vi "server.vi"() -> ()   [LabVIEW 2014, in "Experiment.lvclass"]
uses:
  Experiment.lvclass
  HSDIO/HSDIO_settings.ctl
  <instrlib>/niHSDIO/niHSDIO.llb/niHSDIO_ctl Trigger Script - trigID Values (Ring).ctl
  <instrlib>/niHSDIO/niHSDIO.llb/niHSDIO_ctl Trigger Source Values (Ring).ctl
  <instrlib>/niHSDIO/niHSDIO.llb/niHSDIO_ctl Trigger DigEdge - Edge Values (Ring).ctl
  <instrlib>/niHSDIO/niHSDIO.llb/niHSDIO_ctl Trigger DigLvl - Level Values (Ring).ctl
  HSDIO/waveform.ctl
  Camera/Hamamatsu_C9100-13/camera_setup.ctl
  states.ctl
  Analog_output/AO_settings.ctl
  DAQmx_DO/settings.ctl
  Analog_Input/settings.ctl
  Counter/Counter_Settings_Control.ctl
  <vilib>/Platform/TimedLoop/XDataNode/timing_clust.ctl
  <vilib>/Platform/TimedLoop/XDataNode/nitl_modes.ctl
  <vilib>/Platform/TimedLoop/XDataNode/wakeup.ctl
  Experiment.lvclass/Experiment.ctl
  Globals.vi
  <vilib>/platform/TimedLoop/XDataNode/XDataNode.xnode
  HSDIO/HSDIO.lvclass
  DAQmx_DO/DAQmx_DO.lvclass
  Analog_output/Analog_Output.lvclass
  Analog_Input/Analog_Input.lvclass
  Counter/Counter.lvclass
  Camera/Hamamatsu_C9100-13/Hamamatsu_C9100-13.lvclass
  TCP_IP/TCP_IP.lvclass
  <vilib>/Platform/TimedLoop/XDataNode/XDNodeRunTimeDep.lvlib
panel:
  in  "IP address to listen on\n(blank to allow all networks)":string
  out "cycleContinuously":bool
  out "state":T1
  in  "port":u16=9000
  out "Loops while waiting for measurement isDone?":i32
  out "Log History":string
  in  "Tab Control":T2(tab)
  out "Measurement Timeout (ms)":u32=1
  out "HSDIO Settings":T3={"Enable HSDIO Pulses"=FALSE, "Clock Rate"=20000000.0, "Array of Script Triggers"=[], "Pulse Generation Script"="script script1\n     wait 1\nend script", "Start Trigger"={"Wait for start trigger?"=FALSE, "source (PFI 0)"="PFI0", "edge (rising)"=12, "description"=""}, "Hardware alignment quantum\n(in samples)"=1, "Array of Waveforms"=[], "description"="", "Resource Names"=[], "Active Channels"=[], "Initial States"=[], "Idle States"=[]} {"Hardware alignment quantum\n(in samples)" min=1 step=1; "Array of Script Triggers"."level" items=["High Level"=34, "Low Level"=35]; "Array of Script Triggers"."edge" items=["Rising Edge"=12, "Falling Edge"=13]; "Start Trigger"."edge (rising)" items=["Rising Edge"=12, "Falling Edge"=13]; "Clock Rate" min=0.0 max=200000000.0 format="%.2p"}
  out "Camera Setup":T9={"Analog Gain (0-5)"=0, "Exposure Time"=0.05, "EM Gain (0-255)"=0, "Trigger Polarity"="ATP P", "External Trigger Mode"="EMD L", "Scan Speed"="SSP H", "External Trigger Source"="ESC B", "Scan Mode"="SMD N", "Super Pixel Binning\n(if enabled in Scan Mode)"="1x1", "Camera Sub-array acquisition region\n(if enabled in scan mode)"={"Left"=0, "Top"=0, "Width"=512, "Height"=512}, "Use camera?"=FALSE, "# image buffers"=10, "shots per measurement"=2, "Force images to U16"=FALSE, "Low Light Sensitivity"="LLS 0", "cooling"="CSW F", "fan"="FAN F", "Frame Grabber acquisition region"={"Left"=0, "Top"=0, "Right"=512, "Bottom"=512}} {"Frame Grabber acquisition region"."Bottom" max=512 step=1; "Frame Grabber acquisition region"."Right" max=512 step=1; "Frame Grabber acquisition region"."Top" max=512 step=1; "Frame Grabber acquisition region"."Left" max=512 step=1; "shots per measurement" min=0 step=1; "# image buffers" min=0 step=1; "Camera Sub-array acquisition region\n(if enabled in scan mode)"."Height" min=16 max=512 step=16; "Camera Sub-array acquisition region\n(if enabled in scan mode)"."Width" min=16 max=512 step=16; "Camera Sub-array acquisition region\n(if enabled in scan mode)"."Top" max=496 step=16; "Camera Sub-array acquisition region\n(if enabled in scan mode)"."Left" max=496 step=16; "Analog Gain (0-5)" max=5 step=1}
  out "Analog Output Parameters":T10={"Enable Analog Out?"=FALSE, "Physical Channel"="PXI1Slot2/ao0:2", "Minimum Value"=-10.0, "Maximum Value"=10.0, "Samples per second"=0.0, "Start Trigger"={"Wait for start trigger?"=FALSE, "source"="/Dev1/PFI0", "edge"=10280}, "Analog Output Waveforms (channel, time)"=[], "Export trigger"={"Export Start Trigger?"=FALSE, "output terminal"=""}, "External Clock"={"Use external clock?"=FALSE, "source"="", "max expected clock rate"=200000000.0}} {"External Clock"."max expected clock rate" format="%#_13g"; "Start Trigger"."edge" items=["Rising"=10280, "Falling"=10171]; "Maximum Value" format="%0.2f"; "Minimum Value" format="%0.2f"}
  out "settings":T11={"enable"=FALSE, "samples_per_measurement"=1, "sample rate (Hz)"=-10.0, "source"="Dev3/ai0:2", "Start Trigger"={"Wait for start trigger?"=FALSE, "source"="/Dev1/PFI0", "edge"=10280}, "ground_mode"=""} {"Start Trigger"."edge" items=["Rising"=10280, "Falling"=10171]}
  out "DAQmx Pulse Settings":T12={"Enable DAQmx Pulses"=FALSE, "DAQmx Physical Channels"="Dev2/port0_32", "Clock Rate"=10000000.0, "units/sec (ms=1000)"=1000.0, "Start Trigger"={"Wait for start trigger?"=FALSE, "source"="/Dev1/PFI0", "edge"=10280}, "waveform"={"name"="", "transitions"=[], "states"=[]}} {"Start Trigger"."edge" items=["Rising"=10280, "Falling"=10171]; "Clock Rate" min=0.0 max=200000000.0 format="%.2p"}
  out "Counter Settings":T13 {"Array of Counter Settings"."clock rate (Hz)" format="%0.2f"}
  in  "Clear Log":bool
  in  "Return fake test data":bool
  out "Done":bool=TRUE
  in  "Restart":bool
  out "Log":string
  in  "Stop":bool
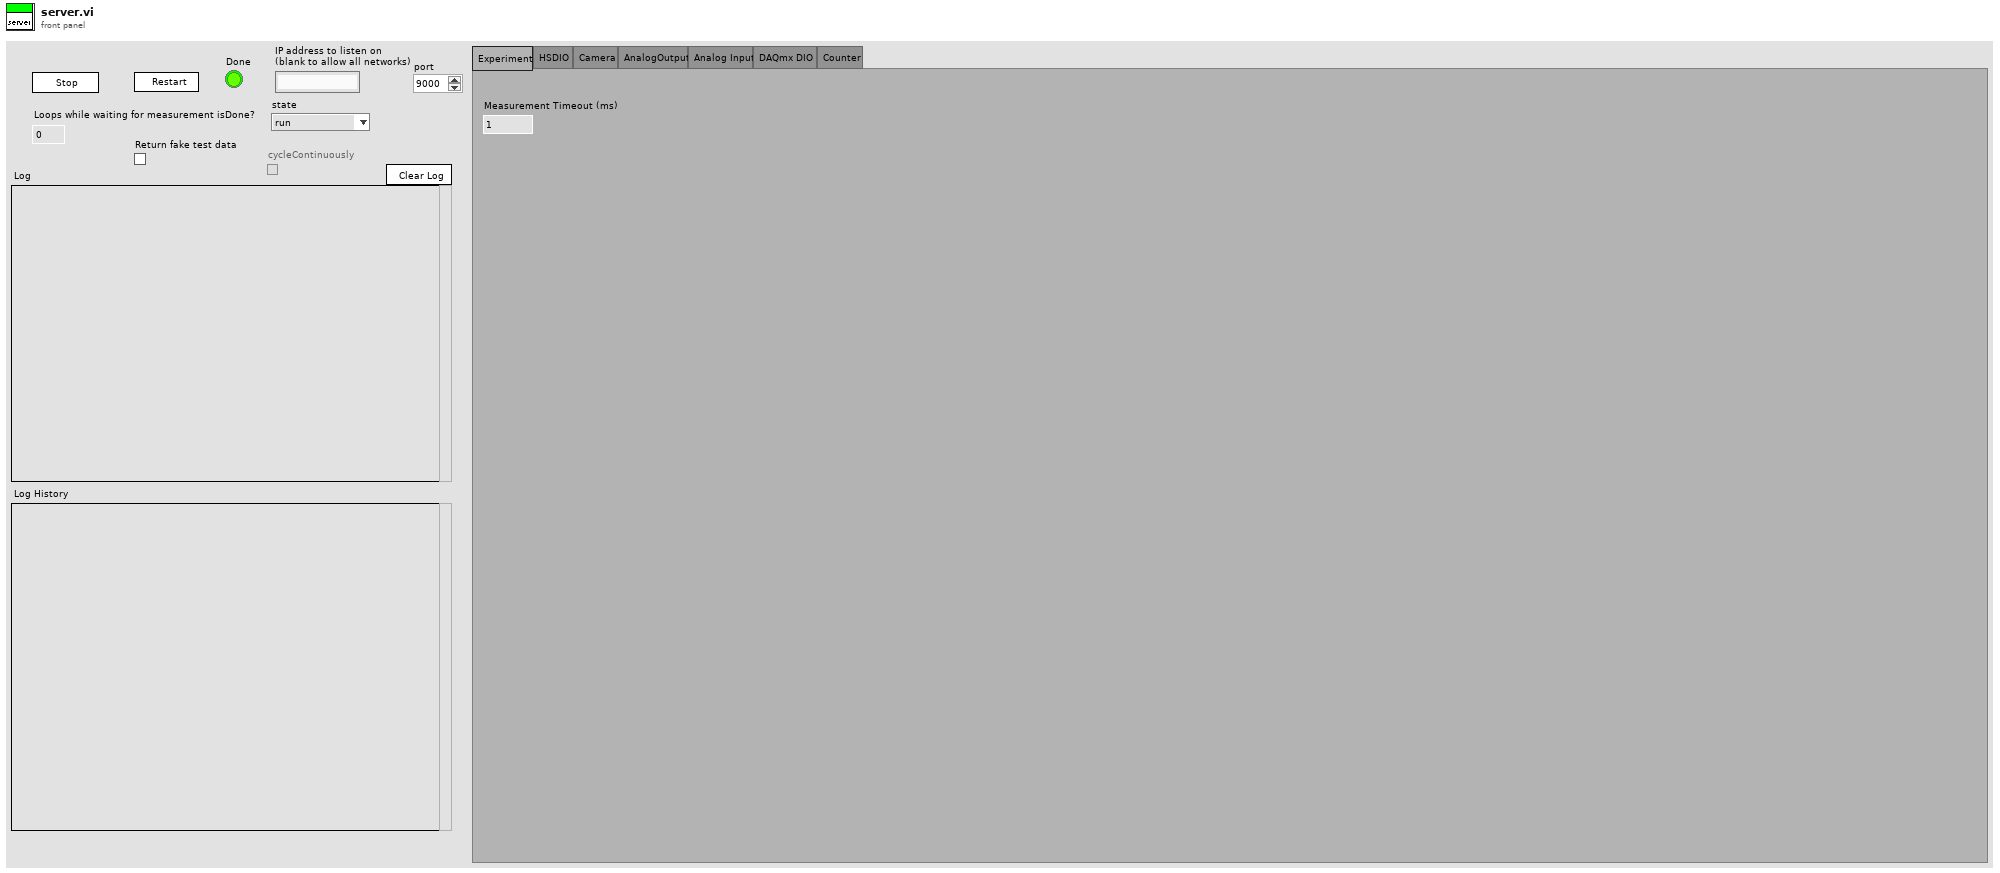
[diagram p1: front panel]
types:
  T1 = typedef "Experiment.lvclass/states.ctl" = enum16{"run", "pause", "shutdown gracefully", "halt immediately", "waiting for connection", "waiting for command"}
  T2 = enum32{"Experiment", "HSDIO", "Camera", "AnalogOutput", "Analog Input", "DAQmx DIO", "Counter"}
  T3 = typedef "HSDIO.lvclass/HSDIO_settings.ctl" = cluster{"Enable HSDIO Pulses":bool, "Clock Rate":dbl, "Array of Script Triggers":cluster{"trigger id (script trigger 0)":T4, "source (PFI 0)":T5, "Trigger Type":enum32{"Edge", "Level"}, "edge":T6, "level":T7}[], "Pulse Generation Script":string, "Start Trigger":cluster{"Wait for start trigger?":bool, "source (PFI 0)":T5, "edge (rising)":T6, "description":string}, "Hardware alignment quantum\n(in samples)":u16, "Array of Waveforms":T8[], "description":string, "Resource Names":refnum<k15>[], "Active Channels":string[], "Initial States":string[], "Idle States":string[]}
  T4 = typedef "niHSDIO_ctl Trigger Script - trigID Values (Ring).ctl" = string
  T5 = typedef "niHSDIO_ctl Trigger Source Values (Ring).ctl" = string
  T6 = typedef "niHSDIO_ctl Trigger DigEdge - Edge Values (Ring).ctl" = i32
  T7 = typedef "niHSDIO_ctl Trigger DigLvl - Level Values (Ring).ctl" = i32
  T8 = typedef "HSDIO.lvclass/waveform.ctl" = cluster{"name":string, "transitions":u32[], "states":u8[][]}
  T9 = typedef "Hamamatsu_C9100-13.lvclass/camera_setup.ctl" = cluster{"Analog Gain (0-5)":u8, "Exposure Time":dbl, "EM Gain (0-255)":u8, "Trigger Polarity":string, "External Trigger Mode":string, "Scan Speed":string, "External Trigger Source":string, "Scan Mode":string, "Super Pixel Binning\n(if enabled in Scan Mode)":string, "Camera Sub-array acquisition region\n(if enabled in scan mode)":cluster{"Left":u16, "Top":u16, "Width":u16, "Height":u16}, "Use camera?":bool, "# image buffers":i32, "shots per measurement":i32, "Force images to U16":bool, "Low Light Sensitivity":string, "cooling":string, "fan":string, "Frame Grabber acquisition region":cluster{"Left":i32, "Top":i32, "Right":i32, "Bottom":i32}}
  T10 = typedef "Analog_Output.lvclass/AO_settings.ctl" = cluster{"Enable Analog Out?":bool, "Physical Channel":tag, "Minimum Value":dbl, "Maximum Value":dbl, "Samples per second":dbl, "Start Trigger":cluster{"Wait for start trigger?":bool, "source":tag, "edge":i32}, "Analog Output Waveforms (channel, time)":dbl[][], "Export trigger":cluster{"Export Start Trigger?":bool, "output terminal":tag}, "External Clock":cluster{"Use external clock?":bool, "source":tag, "max expected clock rate":dbl}}
  T11 = typedef "Analog_Input.lvclass/settings.ctl" = cluster{"enable":bool, "samples_per_measurement":i32, "sample rate (Hz)":dbl, "source":tag, "Start Trigger":cluster{"Wait for start trigger?":bool, "source":tag, "edge":i32}, "ground_mode":string}
  T12 = typedef "DAQmx_DO.lvclass/settings.ctl" = cluster{"Enable DAQmx Pulses":bool, "DAQmx Physical Channels":tag, "Clock Rate":dbl, "units/sec (ms=1000)":dbl, "Start Trigger":cluster{"Wait for start trigger?":bool, "source":tag, "edge":i32}, "waveform":T8}
  T13 = typedef "Counter.lvclass/Counter_Settings_Control.ctl" = cluster{"enable":bool, "Array of Counter Settings":cluster{"counter source":tag, "clock source":tag, "clock rate (Hz)":dbl}[]}
  T14 = typedef "XDNodeRunTimeDep.lvlib/timing_clust.ctl" = cluster{"Expected End [f-1]":u64, "Actual End [f-1]":u64, "Finished Late? [f-1]":bool, "Expected End [i-1]":u64, "Actual End [i-1]":u64, "Finished Late? [i-1]":bool, "Expected Start [i]":u64, "Actual Start [i]":u64, "Expected Start [f]":u64, "Actual Start [f]":u64, "Source Name":string, "Structure Name":string, "Period":i64, "Deadline":i64, "Offset":i64, "Start":i64, "Priority":i32, "Timeout":i32, "Mode":T15, "Wakeup Reason":T16, "Error":errorcluster, "Source Type":string, "Secondary Source Type":string, "Global End Time":u64, "Global Start Time":u64, "Frame Duration":u64, "Iteration Duration":u64, "Assigned CPU":i32, "I/O Scan Engine Mode":u32}
  T15 = typedef "XDNodeRunTimeDep.lvlib/nitl_modes.ctl" = enum32{"No Change", "Process missed periods, maintain original phase", "Discard missed periods, maintain original phase", "Process missed periods, ignore original phase", "Discard missed periods, ignore original phase"}
  T16 = typedef "XDNodeRunTimeDep.lvlib/wakeup.ctl" = enum32{"Normal", "Aborted", "Asynchronous wakeup", "Timing source error", "Timed loop error", "Timeout"}
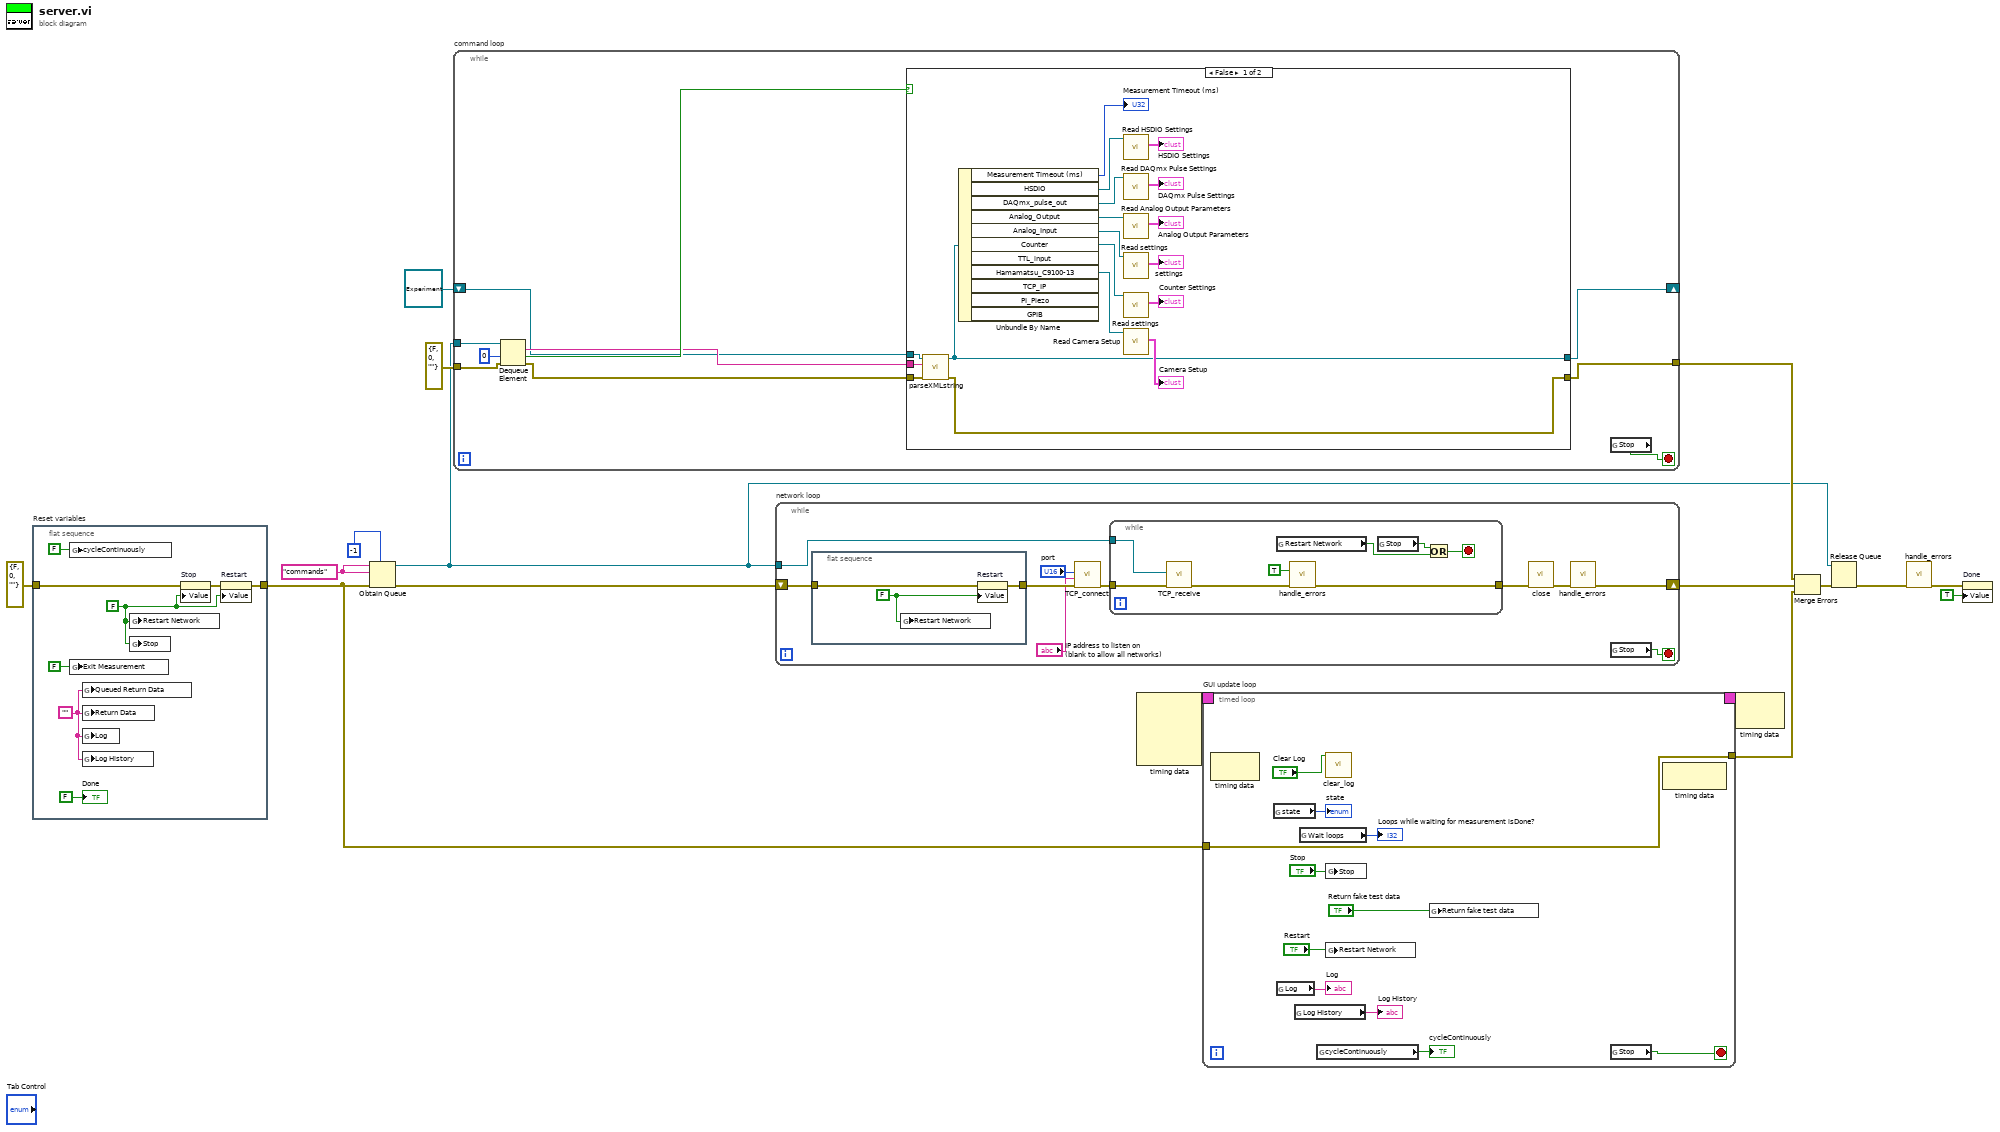
[diagram p0: block diagram]
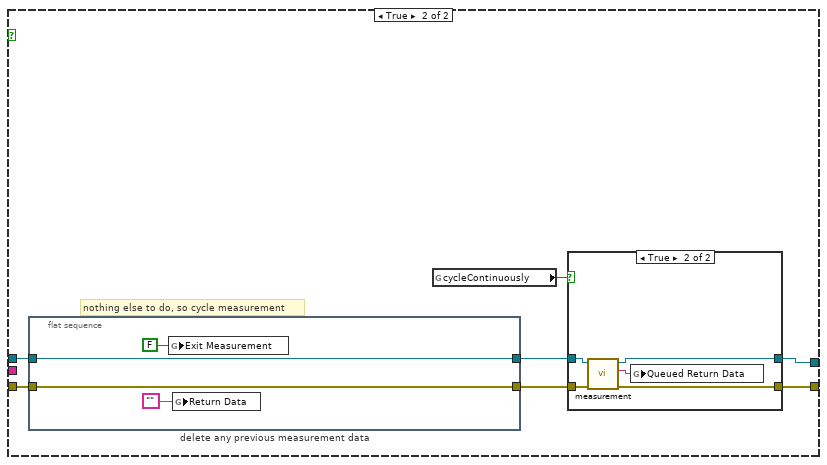
[diagram p2: hidden frame]
diagram:
  w17 = "commands" ("name (unnamed)")
  n1 = flat-sequence "Reset variables" {
    tunnel: [w21] -> w6
    tunnel: errorcluster {"status"=FALSE, "code"=0, "source"=""} ("error in (no error)") -> [w23]
    frame #0 {
      w18 = ""
      w22 = FALSE ("Stop")
      n2 = global write "Globals.vi" "cycleContinuously"(FALSE ("cycle continuously")) -> ()
      n3 = global write "Globals.vi" "Exit Measurement"(FALSE ("Exit Measurement")) -> ()
      n4 = global write "Globals.vi" "Queued Return Data"(w18) -> ()
      n5 = global write "Globals.vi" "Return Data"(w18) -> ()
      n6 = global write "Globals.vi" "Log"(w18) -> ()
      n7 = global write "Globals.vi" "Log History"(w18) -> ()
      n8 = global write "Globals.vi" "Restart Network"(w22) -> ()
      n9 = global write "Globals.vi" "Stop"(w22) -> ()
      n10 = property on="Stop" class="Bool (strict)"(error in=w23, "Value"=w22) -> (error out=w25:errorcluster)  [unwired: 1 in, 1 out]
      n11 = property on="Restart" class="Bool (strict)"(error in=w25, "Value"=w22) -> (error out=w21:errorcluster)  [unwired: 1 in, 1 out]
      "Done" <- FALSE ("Done")
    }
  }
  n12 = Obtain Queue(max queue size (-1, unlimited)=-1, name (unnamed)=w17, element data type=w17, error in (no error)=w6) -> (queue out=w10:refnum<queue>, error out=w16:errorcluster)  [unwired: 1 in, 1 out]
  n13 = while "command loop" {
    tunnel: w10 -> [w35]
    tunnel: errorcluster {"status"=FALSE, "code"=0, "source"=""} ("error constant") -> [w34]
    tunnel: [w26] -> w13
    shift-right: [w28] -> _
    shift-left: refnum<class "Experiment.lvclass"> refnum ("Experiment.lvclass") -> [w29]
    stop <- w27 stop-if-true
    n14 = Dequeue Element(queue=w35, timeout in ms (-1)=0, error in (no error)=w34) -> (element=w31:string, timed out?=w32:bool, error out=w33:errorcluster)  [unwired: 1 out]
    n15 = case shown="False" w32 {
      tunnel: [w53 w59] -> w26
      tunnel: w33 -> [w50 w56]
      tunnel: w31 -> [w52 _]
      tunnel: w29 -> [w51 w54]
      tunnel: [w45 w58] -> w28
      frame False {
        n16 = call "parseXMLstring.vi"("error in (no error)"=w50, "Node Value"=w52, "Experiment.lvclass (in)"=w51) -> ("error out"=w53:errorcluster, "Experiment.lvclass"=w45:refnum<class "Experiment.lvclass">)  [unwired: 7 in]
        n17 = Unbundle By Name(w45) -> ("Measurement Timeout (ms)"=→"Measurement Timeout (ms)":u32, "HSDIO"=w49:refnum<class "HSDIO.lvclass">, "DAQmx_pulse_out"=w42:refnum<class "DAQmx_DO.lvclass">, "Analog_Output"=w44:refnum<class "Analog_Output.lvclass">, "Analog_Input"=w39:refnum<class "Analog_Input.lvclass">, "Counter"=w37:refnum<class "Counter.lvclass">, "Hamamatsu_C9100-13"=w47:refnum<class "Hamamatsu_C9100-13.lvclass">)  [unwired: 4 out]
        n18 = call-dynamic "Read HSDIO Settings.vi"("HSDIO in"=w49) -> ("HSDIO Settings"=→"HSDIO Settings":T3)  [unwired: 5 in, 5 out]
        n19 = call-dynamic "Read DAQmx Pulse Settings.vi"("DAQmx_pulse_out in"=w42) -> ("DAQmx Pulse Settings"=→"DAQmx Pulse Settings":T12)  [unwired: 10 in]
        n20 = call-dynamic "Read Analog Output Parameters.vi"("Analog_Output in"=w44) -> ("Analog Output Parameters"=→"Analog Output Parameters":T10)  [unwired: 8 in, 2 out]
        n21 = call-dynamic "Read settings.vi"("Analog_Input in"=w39) -> ("settings"=→"settings":T11)  [unwired: 8 in, 2 out]
        n22 = call-dynamic "Read settings.vi"("Counter in"=w37) -> ("Counter Settings"=→"Counter Settings":T13)  [unwired: 8 in, 2 out]
        n23 = call-dynamic "Read Camera Setup.vi"("Hamamatsu_C9100-13 in"=w47) -> ("Camera Setup"=→"Camera Setup":T9)  [unwired: 8 in, 2 out]
      }
      frame True {
        # "nothing else to do, so cycle measurement"
        n24 = flat-sequence "delete any previous measurement data" {
          tunnel: [w63] -> w57
          tunnel: w56 -> [w63]
          tunnel: [w62] -> w55
          tunnel: w54 -> [w62]
          frame #0 {
            n25 = global write "Globals.vi" "Exit Measurement"(FALSE ("Exit Measurement")) -> ()
            n26 = global write "Globals.vi" "Return Data"("") -> ()
          }
        }
        n27 = global read "Globals.vi" "cycleContinuously"() -> (w60:bool)
        n28 = case shown="True" w60 {
          tunnel: w57 -> [w65 w71]
          tunnel: [w65 w70] -> w59
          tunnel: w55 -> [w66 w69]
          tunnel: [w66 w68] -> w58
          frame False {
          }
          frame True {
            n29 = call "measurement.vi"("error in (no error)"=w71, "Experiment.lvclass"=w69) -> ("error out"=w70:errorcluster, "returndata"=w67:string, "Experiment out"=w68:refnum<class "Experiment.lvclass">)  [unwired: 5 in]
            n30 = global write "Globals.vi" "Queued Return Data"(w67) -> ()
          }
        }
      }
    }
    n31 = global read "Globals.vi" "Stop"() -> (w27:bool)
  }
  n32 = while "network loop" {
    shift-right: [w81] -> w9
    shift-left: w16 -> [w74]
    tunnel: w10 -> [w80]
    stop <- w78 stop-if-true
    n33 = flat-sequence {
      tunnel: [w83] -> w75
      tunnel: w74 -> [w84]
      frame #0 {
        w82 = FALSE ("Restart")
        n34 = global write "Globals.vi" "Restart Network"(w82) -> ()
        n35 = property on="Restart" class="Bool (strict)"(error in=w84, "Value"=w82) -> (error out=w83:errorcluster)  [unwired: 1 in, 1 out]
      }
    }
    n36 = call "TCP_connect.vi"("error in (no error)"=w75, "IP address to listen on\n(blank to allow all networks)"="IP address to listen on\n(blank to allow all networks)", "port"="port") -> ("error out"=w76:errorcluster)  [unwired: 8 in]
    n37 = while {
      tunnel: w76 -> [w90]
      tunnel: [w92] -> w79
      tunnel: w80 -> [w91]
      stop <- w89 stop-if-true
      n38 = call "TCP_receive.vi"("error in (no error)"=w90, "queue"=w91) -> ("error out"=w86:errorcluster)  [unwired: 9 in]
      n39 = global read "Globals.vi" "Restart Network"() -> (w87:bool)
      n40 = call "handle_errors.vi"("Restart Network"=TRUE, "error in (no error)"=w86) -> ("error out"=w92:errorcluster)  [unwired: 13 in]
      n41 = global read "Globals.vi" "Stop"() -> (w88:bool)
      n42 = Or(x=w88, y=w87) -> (x .or. y?=w89:bool)
    }
    n43 = call "close.vi"("error in (no error)"=w79) -> ("error out"=w77:errorcluster)  [unwired: 10 in]
    n44 = call "handle_errors.vi"("error in (no error)"=w77) -> ("error out"=w81:errorcluster)  [unwired: 14 in]
    n45 = global read "Globals.vi" "Stop"() -> (w78:bool)
  }
  n46 = node-c288() -> (w2:T14)  [unwired: 4 in]
  n47 = timed-loop "GUI update loop" {
    tunnel: w6 -> [w99]
    tunnel: [w99] -> w5
    timing: w2 -> [_]
    timing-out: [_] -> w1
    stop <- w100 stop-if-true
    n48 = node-c288() -> ()  [unwired: 1 in, 1 out]
    n49 = global read "Globals.vi" "state"() -> (→"state":T1)
    n50 = global read "Globals.vi" "Log"() -> (→"Log":string)
    n51 = global read "Globals.vi" "Log History"() -> (→"Log History":string)
    n52 = global read "Globals.vi" "Wait loops"() -> (→"Loops while waiting for measurement isDone?":i32)
    n53 = global read "Globals.vi" "cycleContinuously"() -> (→"cycleContinuously":bool)
    n54 = call "clear_log.vi"("clear log?"="Clear Log") -> ()  [unwired: 10 in, 1 out]
    n55 = global write "Globals.vi" "Stop"("Stop") -> ()
    n56 = global write "Globals.vi" "Restart Network"("Restart") -> ()
    n57 = global write "Globals.vi" "Return fake test data"("Return fake test data") -> ()
    n58 = global read "Globals.vi" "Stop"() -> (w100:bool)
    n59 = node-c288() -> ()  [unwired: 1 in, 1 out]
  }
  n60 = node-c288(w1) -> ()  [unwired: 1 out]
  n61 = Merge Errors(w13, w9, w5) -> (w12:errorcluster)
  n62 = Release Queue(queue=w10, error in (no error)=w12) -> (error out=w11:errorcluster)  [unwired: 1 in, 2 out]
  n63 = call "handle_errors.vi"("error in (no error)"=w11) -> ("error out"=w4:errorcluster)  [unwired: 14 in]
  n64 = property on="Done" class="Bool (strict)"(error in=w4, "Value"=TRUE ("Done")) -> ()  [unwired: 1 in, 2 out]
